vi "DigitalSourceToValue.vi"(1 "AnalogTriggers":bool[](array[boolean])=[FALSE, FALSE, FALSE, FALSE, FALSE, FALSE, FALSE, FALSE], 2 "DigitalInputs":bool[](array[boolean])=[FALSE, FALSE, FALSE, FALSE, FALSE, FALSE, FALSE, FALSE, FALSE, FALSE, FALSE, FALSE, FALSE, FALSE, FALSE, FALSE, FALSE, FALSE, FALSE, FALSE, FALSE, FALSE, FALSE, FALSE, FALSE, FALSE], 3 "Source":T1) -> (0 "Value":bool)   [LabVIEW 2019]
uses:
  Source.ctl
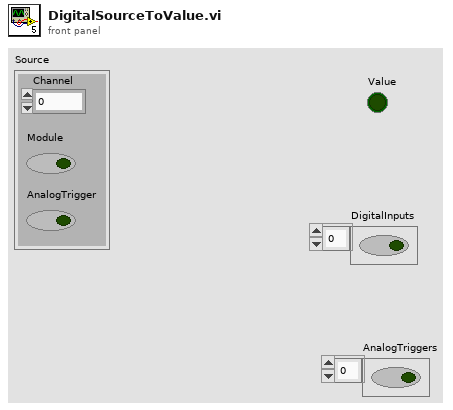
[diagram p1: front panel]
types:
  T1 = typedef "Source.ctl" = cluster{"Channel":fxp<+,4,4>, "Module":bool, "AnalogTrigger":bool}
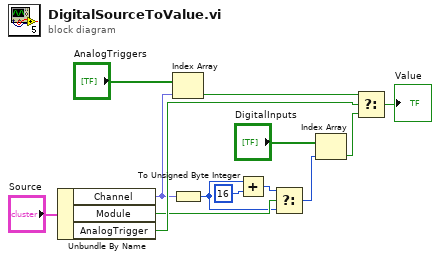
[diagram p0: block diagram]
diagram:
  n1 = Unbundle By Name("Source") -> ("Channel"=w6:fxp<+,4,4>, "Module"=w8:bool, "AnalogTrigger"=w12:bool)
  n2 = Index Array(array="AnalogTriggers", index=w6) -> (element=w10:bool)
  n3 = To Unsigned Byte Integer(number=w6) -> (unsigned 8bit integer=w4:u8)
  n4 = Add(x=w4, y=u8 16) -> (x+y=w7:u8)
  n5 = Select(t=w7, s=w8, f=w4) -> (s? t:f=w2:u8)
  n6 = Index Array(array="DigitalInputs", index=w2) -> (element=w1:bool)
  n7 = Select(t=w10, s=w12, f=w1) -> (s? t:f=→"Value":bool)
